vi "BK Precision 169XB Output DC Volts.vi"() -> ()   [LabVIEW 2021]
doc: "This example shows how to configure the instrument's output voltage level, over current protection, and over voltage protection. The actual voltage level and actual current level are returned as well as whether over voltage protection (OVP) or over current protection (OCP) has been tripped."
uses:
  BK Precision 169XB.lvlib
panel:
  out "Elapsed Time (s)":dbl
  in  "Set Voltage":dbl format="%.1g"
  in  "Set Current":dbl format="%.1g"
  in  "SOVP":dbl format="%0.1f"
  in  "Stop Output":bool
  out "CC Mode?":bool
  out "Actual Current Limit (A)":dbl format="%.2f"
  out "Actual Voltage Level (V)":dbl format="%.2f"
  in  "VISA resource name":refnum<visa-resource-name>
  # "(c) 2014 <Enter Company Name Here>.  ALL RIGHTS RESERVED."
  # "Over Voltage Protection"
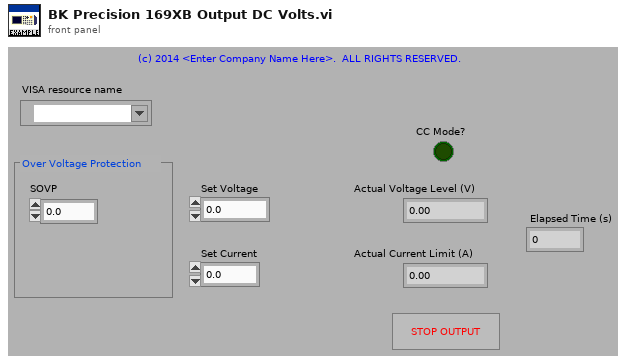
[diagram p1: front panel]
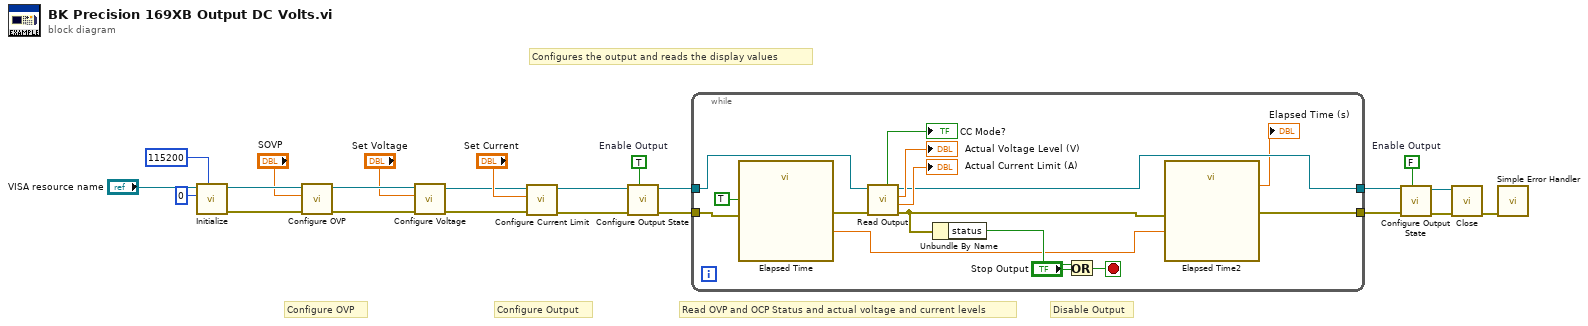
[diagram p0: block diagram]
diagram:
  w13 = FALSE  # Enable Output
  w14 = TRUE  # Enable Output
  # "Configures the output and reads the display values"
  # "Disable Output"
  # "Read OVP and OCP Status and actual voltage and current levels"
  # "Configure Output"
  # "Configure OVP"
  n1 = call "Initialize.vi"("baud rate (9600)"=u32 115200, "Address"=u32 0, "VISA resource name"="VISA resource name") -> ("error out"=w10:errorcluster, "VISA resource name out"=w11:refnum<visa-resource-name>)  [unwired: 7 in]
  n2 = call "Configure OVP.vi"("error in (no error)"=w10, "SOVP"="SOVP", "VISA resource name"=w11) -> ("error out"=w6:errorcluster, "VISA resource name out"=w7:refnum<visa-resource-name>)  [unwired: 7 in]
  n3 = call "Configure Voltage.vi"("error in (no error)"=w6, "Set Voltage"="Set Voltage", "VISA resource name"=w7) -> ("error out"=w5:errorcluster, "VISA resource name out"=w4:refnum<visa-resource-name>)  [unwired: 7 in]
  n4 = call "Configure Current Limit.vi"("error in (no error)"=w5, "Set Current"="Set Current", "VISA resource name"=w4) -> ("error out"=w21:errorcluster, "VISA resource name out"=w22:refnum<visa-resource-name>)  [unwired: 7 in]
  n5 = call "Configure Output State.vi"("Enable Output (T: Enable)"=w14, "error in (no error)"=w21, "VISA resource name"=w22) -> ("error out"=w19:errorcluster, "VISA resource name out"=w20:refnum<visa-resource-name>)  [unwired: 7 in]
  n6 = while {
    tunnel: w20 -> [w25]
    tunnel: [w26] -> w18
    tunnel: w19 -> [w32]
    tunnel: [w27] -> w17
    stop <- w36 stop-if-true
    n7 = call "Elapsed Time"("Auto Reset"=TRUE, "error in (no error)"=w32) -> ("Get Start Time (s)"=w29:dbl, "error out"=w31:errorcluster)  [unwired: 10 in, 6 out]
    n8 = call "Read Output.vi"("error in (no error)"=w31, "VISA resource name"=w25) -> ("error out"=w28:errorcluster, "Current"=→"Actual Current Limit (A)":dbl, "Voltage"=→"Actual Voltage Level (V)":dbl, "VISA resource name out"=w26:refnum<visa-resource-name>, "CC Mode"=→"CC Mode?":bool)  [unwired: 5 in]
    n9 = Unbundle By Name(w28) -> ("status"=w34:bool)
    n10 = Or(x=w34, y="Stop Output") -> (x .or. y?=w36:bool)
    n11 = call "Elapsed Time2"("error in (no error)"=w28, "Set Start Time (s)"=w29) -> ("Elapsed Time (s)"=→"Elapsed Time (s)":dbl, "error out"=w27:errorcluster)  [unwired: 10 in, 6 out]
  }
  n12 = call "Configure Output State.vi"("Enable Output (T: Enable)"=w13, "error in (no error)"=w17, "VISA resource name"=w18) -> ("error out"=w15:errorcluster, "VISA resource name out"=w16:refnum<visa-resource-name>)  [unwired: 7 in]
  n13 = call "Close.vi"("error in (no error)"=w15, "VISA resource name"=w16) -> ("error out"=w12:errorcluster)  [unwired: 9 in]
  n14 = call <vilib>:"Simple Error Handler.vi"("error in (no error)"=w12) -> ()  [unwired: 4 in, 5 out]
